vi "WilliamPI_CameraSend Images To PC Loop2.vi"(8 "error in (no error)":errorcluster, 11 "CameraDevRef":T1) -> ()   [LabVIEW 2015]
doc: "This VI is used to send images to the dashboard using the second enet port on the 8 slot controller. This is provided for compatibility, but is higher overhead than using the Camera MJPG approach.\n\nThis software is licensed. Open the labview\\readme\\WPI Robotics Library Open Source License.txt file for more information."
uses:
  <vilib>/Rock Robotics/WPI/Camera/WPI_CameraDevRef.ctl
  <vilib>/Rock Robotics/SystemInterfaces/NetworkCommunication/NetComm_UsageReport_ResourceType.ctl
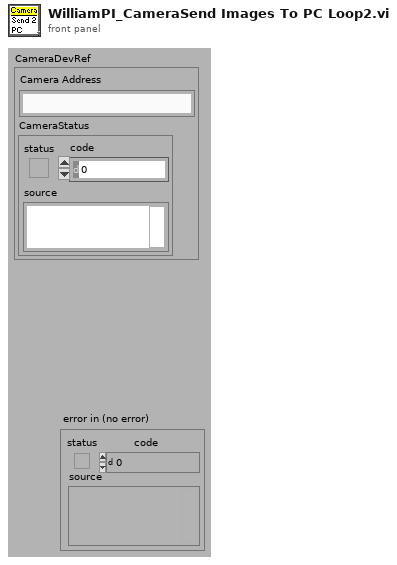
[diagram p1: front panel]
types:
  T1 = typedef "WPI_CameraDevRef.ctl" = cluster{"Camera Address":string, "CameraStatus":errorcluster}
  T2 = cluster{"fps":i32, "compression":i32, "compression 2":i32}
  T3 = typedef "NetComm_UsageReport_ResourceType.ctl" = enum8{"Controller", "Module", "Language", "CANPlugin", "Accelerometer", "ADXL345", "AnalogChannel", "AnalogTrigger", "AnalogTriggerOutput", "CANJaguar", "Compressor", "Counter", "Dashboard", "DigitalInput", "DigitalOutput", "DriverStationCIO", "DriverStationEIO", "DriverStationLCD", "Encoder", "GearTooth", "Gyro", "I2C", "Framework", "Jaguar", "Joystick", "Kinect", "KinectStick", "PIDController", "Preferences", "PWM", "Relay", "RobotDrive", "SerialPort", "Servo", "Solenoid", "SPI", "Task", "Ultrasonic", "Victor", "Button", "Command", "AxisCamera", "PCVideoServer", "SmartDashboard", "Talon", "HiTechnicColorSensor", "HiTechnicAccel", "HiTechnicCompass", "SRF08", "AnalogOutput", "Victor SP", "Talon SRX", "CAN Talon SRX", "ADXL362 Accel", "ADXRS450 Gyro", "Rev SPARK", "Mindsensors SD540", "Digital Filter"}
  T4 = enum16{"Update Mode", "Get Image", "Get Image Data"}
  T5 = typedef "Image Type" = u32
  T6 = typedef "IMAQ Image.ctl" = refnum<image>
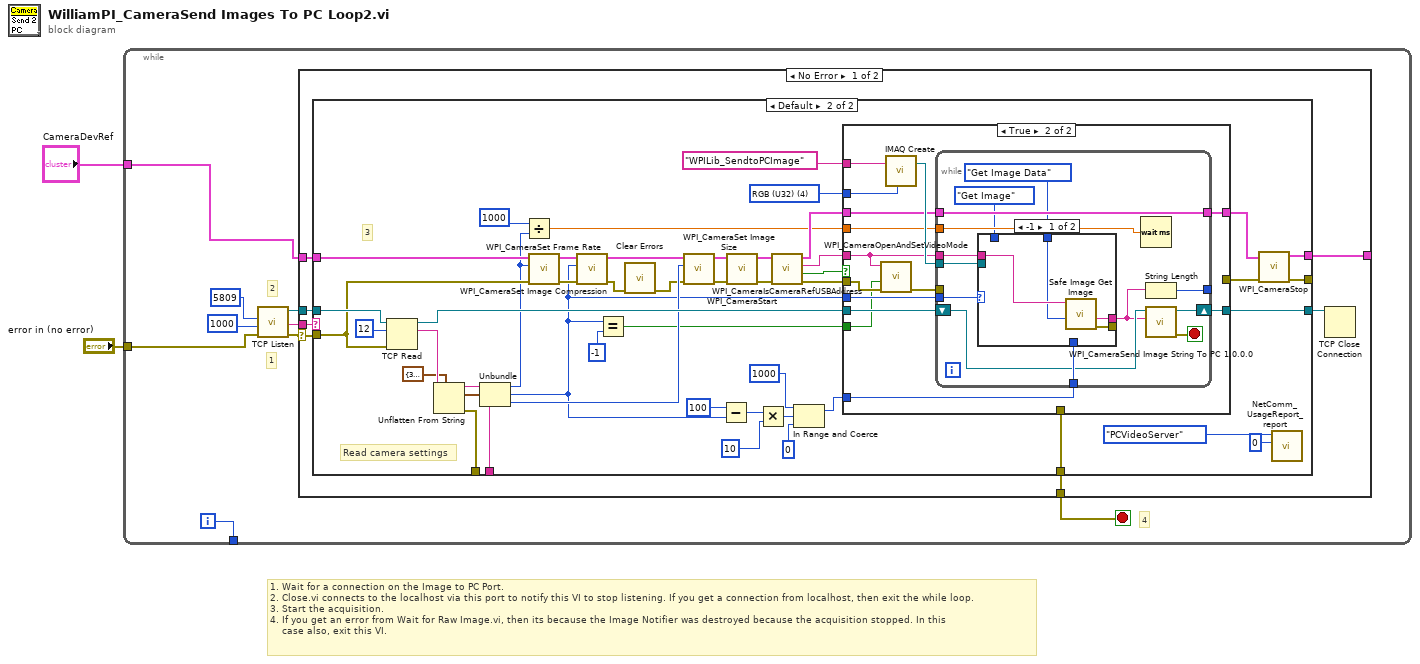
[diagram p0: block diagram]
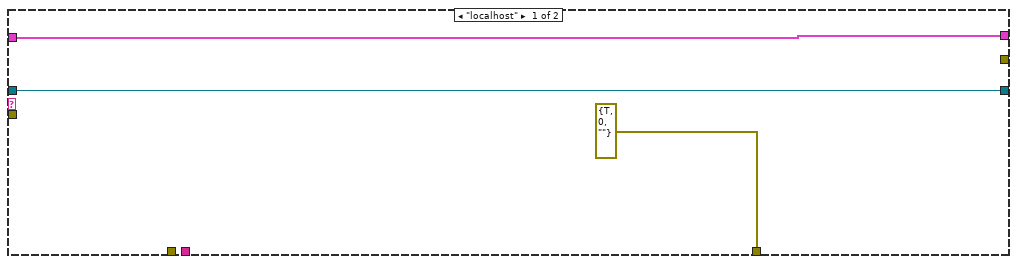
[diagram p2: hidden frame]
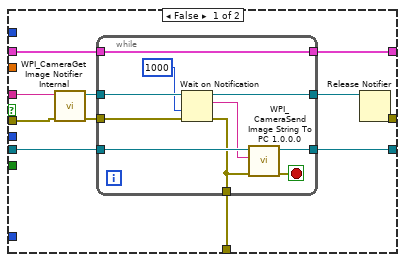
[diagram p3: hidden frame]
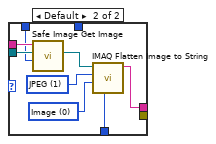
[diagram p4: hidden frame]
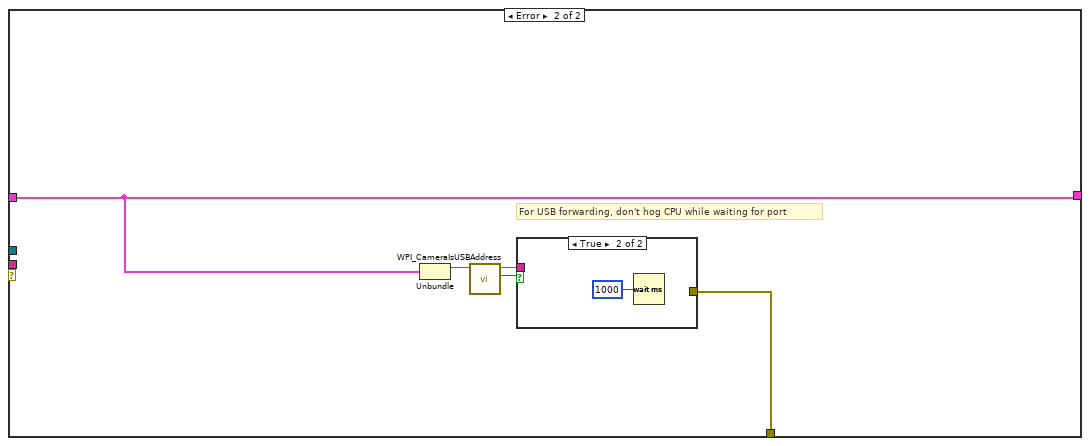
[diagram p5: hidden frame]
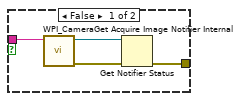
[diagram p6: hidden frame]
diagram:
  # "1. Wait for a connection on the Image to PC Port.\n2. Close.vi connects to the localhost via this port to notify this VI to stop listening. If you get a connection from localhost, then exit the while loop.\n3. Start the acquisition.\n4. If you get an error from Wait for Raw Image.vi, then its because the Image Notifier was destroyed because the acquisition stopped. In this\n    case also, exit this VI."
  n1 = while {
    tunnel: "error in (no error)" -> [w10]
    tunnel: [w4] -> _
    tunnel: "CameraDevRef" -> [w3]
    i -> [w4]
    stop <- w8 stop-if-true
    # "4"
    # "1"
    # "2"
    n2 = call <vilib>:"TCP Listen.vi"("error in (no error)"=w10, "timeout ms (wait forever: -1)"=u16 1000 ("port"), "port"=u16 5809) -> ("error out"=w6:errorcluster, "remote address"=w11:string, "connection ID"=w9:refnum<k5>)  [unwired: 1 in, 5 out]
    n3 = case shown="No Error" w6 {
      selector: w6 -> [w12 _]
      tunnel: [w18 w132] -> _
      tunnel: w11 -> [w17 _]
      tunnel: w3 -> [w16 w132]
      tunnel: w9 -> [w15 _]
      tunnel: [w14 w133] -> w8
      frame No Error {
        n4 = case shown="Default" w17 {
          tunnel: [w21 w66] -> w18
          tunnel: w16 -> [w21 w48]
          tunnel: w12 -> [_ w44]
          tunnel: w15 -> [w19 w52]
          tunnel: [errorcluster {"status"=TRUE, "code"=0, "source"=""} ("error out 2") w68] -> w14
          tunnel: [w19 w67] -> w13
          tunnel: [_ w65] -> _
          tunnel: [_ w23] -> _
          tunnel: [_ w22] -> _
          frame "localhost" {
          }
          frame Default {
            w59 = T5 4 items=["Grayscale (U8)", "Grayscale (I16)", "Grayscale (SGL)", "Complex (CSG)", "RGB (U32)", "HSL (U32)", "RGB (U64)", "Grayscale (U16)"] ("Image Type")
            # "Read camera settings"
            # "3"
            n5 = TCP Read(connection ID=w52, bytes to read=12, error in (no error)=w44) -> (connection ID out=w51:refnum<k5>, data out=w49:string)  [unwired: 2 in, 1 out]
            n6 = Unflatten From String(type=T2 {"fps"=30, "compression"=32, "compression 2"=32} ("Camera Settings"), binary string=w49) -> (rest of the binary string=w22:string, value=w41:T2, error out=w23:errorcluster)  [unwired: 3 in]
            n7 = Unbundle(w41) -> ("fps"=w38:i32, "compression"=w27:i32, "compression 2"=w40:i32)
            n8 = Divide(x=u16 1000 ("port"), y=w38) -> (x/y=w37:dbl)
            n9 = call <vilib>:"WPI_CameraSet Frame Rate.vi"("error in (no error)"=w44, "Frame Rate (fps)"=w38, "CameraDevRef"=w48) -> ("error out"=w43:errorcluster, "CameraDevRef Out"=w47:T1)  [unwired: 7 in]
            n10 = call <vilib>:"WPI_CameraSet Image Compression.vi"("error in (no error)"=w43, "Compression"=w27, "CameraDevRef"=w47) -> ("error out"=w25:errorcluster, "CameraDevRef Out"=w46:T1)  [unwired: 7 in]
            n11 = Equal?(x=w27, y=-1) -> (x = y?=w26:bool)
            n12 = call <vilib>:"Clear Errors.vi"("error in (no error)"=w25) -> ("error out"=w24:errorcluster)  [unwired: 5 in, 1 out]
            n13 = call <vilib>:"WPI_CameraSet Image Size.vi"("error in (no error)"=w24, "Image Size"=w40, "CameraDevRef"=w46) -> ("error out"=w42:errorcluster, "CameraDevRef Out"=w45:T1)  [unwired: 7 in]
            n14 = Subtract(x=100, y=w27) -> (x-y=w32:i32)
            n15 = call <vilib>:"WPI_CameraStart.vi"("error in (no error)"=w42, "CameraDevRef"=w45) -> ("error out"=w56:errorcluster, "CameraDevRef"=w54:T1)  [unwired: 8 out]
            n16 = Multiply(x=w32, y=10) -> (x*y=w34:i32)
            n17 = call <vilib>:"WPI_CameraIsCameraRefUSBAddress.vi"("error in (no error)"=w56, "CameraDevRef"=w54) -> ("error out"=w55:errorcluster, "USB?"=w57:bool, "Camera Address Out"=w58:string, "CameraDevRef out"=w53:T1)  [unwired: 6 in]
            n18 = In Range and Coerce(upper limit=1000, x=w34, lower limit=0) -> (coerced(x)=w30:i32)  [unwired: 1 out]
            n19 = case shown="True" w57 {
              tunnel: w51 -> [w79 w103]
              tunnel: [w78 _] -> w68
              tunnel: [w77 w102] -> w67
              tunnel: w55 -> [w76 w93]
              tunnel: w58 -> [w74 w92]
              tunnel: [w73 w97] -> w64
              tunnel: w53 -> [w72 w98]
              tunnel: [w70 _] -> w63
              tunnel: "WPILib_SendtoPCImage" -> [_ w100]
              tunnel: w59 -> [_ w99]
              tunnel: w30 -> [_ w96]
              tunnel: w37 -> [_ w95]
              tunnel: w27 -> [_ w94]
              tunnel: w26 -> [_ w90]
              frame False {
                n20 = call <vilib>:"WPI_CameraGet Image Notifier Internal.vi"("error in (no error)"=w76, "Camera Address"=w74) -> ("error out"=w75:errorcluster, "Image Notifier"=w71:refnum<notifier>)  [unwired: 8 out]
                n21 = while {
                  tunnel: w75 -> [w85]
                  tunnel: w79 -> [w89]
                  tunnel: [w82] -> w78
                  tunnel: [w87] -> w77
                  tunnel: [w86] -> w73
                  tunnel: w72 -> [w86]
                  tunnel: w71 -> [w84]
                  tunnel: [w80] -> w69
                  stop <- w88 stop-if-true
                  n22 = Wait on Notification(notifier=w84, timeout in ms (-1)=1000 ("Timeout in ms (-1)"), error in (no error)=w85) -> (notifier out=w80:refnum<notifier>, notification=w83:string, error out=w82:errorcluster)  [unwired: 2 out]
                  n23 = call <vilib>:"WPI_CameraSend Image String To PC 1.0.0.0.vi"("error in (no error)"=w82, "String"=w83, "TCP Connection ID"=w89) -> ("error out"=w88:errorcluster, "TCP Connection ID out"=w87:refnum<k5>)  [unwired: 7 out]
                }
                n24 = Release Notifier(notifier=w69) -> (error out=w70:errorcluster)  [unwired: 1 in, 3 out]
              }
              frame True {
                n25 = call <vilib>:"WPI_CameraOpenAndSetVideoMode.vi"("error in (no error)"=w93, "USB JPEG"=w90, "Camera Address Out"=w92) -> ("error out"=w91:errorcluster)  [unwired: 8 in]
                n26 = call "IMAQ Create"("Image Name"=w100, "Image Type"=w99) -> ("New Image"=w101:T6)  [unwired: 3 in, 1 out]
                n27 = while {
                  tunnel: w92 -> [w115]
                  shift-right: [w116] -> w102
                  shift-left: w103 -> [w109]
                  tunnel: w101 -> [w114]
                  tunnel: [w112] -> w97
                  tunnel: w98 -> [w112]
                  tunnel: w96 -> [w111]
                  tunnel: w95 -> [w110]
                  tunnel: [w107] -> _
                  tunnel: w94 -> [w106]
                  tunnel: w91 -> [_]
                  stop <- w113 stop-if-true
                  n28 = case shown="-1" w106 {
                    tunnel: [w119 w128] -> w108
                    tunnel: w115 -> [w120 w124]
                    tunnel: w114 -> [_ w123]
                    tunnel: w111 -> [_ w125]
                    tunnel: [w118 _] -> _
                    tunnel: T4."Get Image Data" ("Operation") -> [w117 _]
                    tunnel: T4."Get Image" ("Operation") -> [_ w121]
                    frame -1 {
                      n29 = call <vilib>:"Safe Image Get Image.vi"("Operation"=w117, "Session In"=w120) -> ("error out"=w118:errorcluster, "Image Data String"=w119:string)  [unwired: 6 in, 2 out]
                    }
                    frame Default {
                      w126 = 0 items=["Image", "Image and Vision Info", "Reference to Image"] ("Type of Flatten (Image and Vision Info)")
                      w127 = 1 items=["None", "JPEG", "PACKED BINARY"] ("Compression (None)")
                      n30 = call <vilib>:"Safe Image Get Image.vi"("Operation"=w121, "Image In"=w123, "Session In"=w124) -> ("Image Out"=w122:T6)  [unwired: 5 in, 3 out]
                      n31 = call "IMAQ Flatten Image to String"("Quality (750)"=w125, "Type of Flatten (Image and Vision Info)"=w126, "Compression (None)"=w127, "Image"=w122) -> ("Data String"=w128:string)  [unwired: 6 in, 1 out]
                    }
                  }
                  n32 = Wait (ms)(milliseconds to wait=w110) -> ()  [unwired: 1 out]
                  n33 = String Length(string=w108) -> (length=w107:i32)
                  n34 = call <vilib>:"WPI_CameraSend Image String To PC 1.0.0.0.vi"("String"=w108, "TCP Connection ID"=w109) -> ("error out"=w113:errorcluster, "TCP Connection ID out"=w116:refnum<k5>)  [unwired: 1 in, 7 out]
                }
              }
            }
            n35 = call <vilib>:"WPI_CameraStop.vi"("error in (no error)"=w63, "CameraDevRef"=w64) -> ("error out"=w65:errorcluster, "CameraDevRef"=w66:T1)  [unwired: 8 out]
            n36 = call <vilib>:"NetComm_UsageReport_report.vi"("Instance Number"=u8 0, "Resource Type"=NetComm_UsageReport_ResourceType."PCVideoServer") -> ()  [unwired: 10 in]
          }
        }
        n37 = TCP Close Connection(connection ID=w13) -> ()  [unwired: 1 in, 3 out]
      }
      frame Error {
        # "For USB forwarding, don't hog CPU while waiting for port"
        n38 = Unbundle(w132) -> ("Camera Address"=w131:string)  [unwired: 1 out]
        n39 = call <vilib>:"WPI_CameraIsUSBAddress.vi"("Camera Address In"=w131) -> ("USB?"=w129:bool, "Camera Address Out"=w130:string)  [unwired: 8 in, 1 out]
        n40 = case shown="True" w129 {
          tunnel: [w137 _] -> w133
          tunnel: w130 -> [w134 _]
          frame False {
            n41 = call <vilib>:"WPI_CameraGet Acquire Image Notifier Internal.vi"("Camera Address"=w134) -> ("error out"=w135:errorcluster, "Acquire Image Notifier"=w136:refnum<notifier>)  [unwired: 1 in, 8 out]
            n42 = Get Notifier Status(notifier=w136, error in (no error)=w135) -> (error out=w137:errorcluster)  [unwired: 4 out]
          }
          frame True {
            n43 = Wait (ms)(milliseconds to wait=u32 1000) -> ()  [unwired: 1 out]
          }
        }
      }
    }
  }
